vi "PH_ImageOperator.Best GAUSS Procedure.vi"(1 "Diameter":dbl, 2 "Data Trace":cluster{"Index":sgl[], "Trace":sgl[]}, 3 "calibrated?":bool, 4 "No Offset?":bool, 5 "error in (no error)":errorcluster) -> (16 "Best Fit Trace":cluster{"Index":sgl[], "Best Fit":dbl[]}, 17 "Best Fit Width Parameter":dbl, 18 "Best Fit Order":i32, 19 "error out":errorcluster)   [LabVIEW 2014, in "PH_ImageOperator.lvlib"]
doc: "Within this VI a GAUSS fit routine up to the 20th order is called and applied to the \"Data Trace\" (the Diameter\" is used within the fit routine as start value). The loop is stopped if the 10th order is reached or the mean square error increases. The error is caused by the fit routine only. If \"No Offset\" is true, within the fit function no offset is assumed."
uses:
  PH_ImageOperator.lvlib
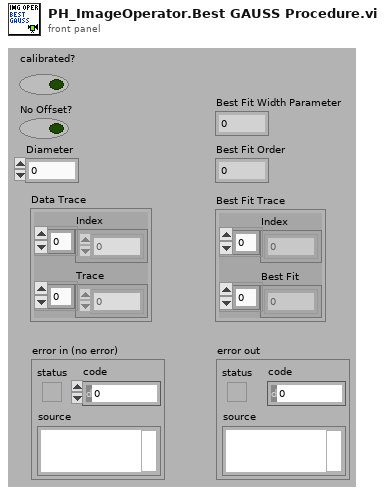
[diagram p1: front panel]
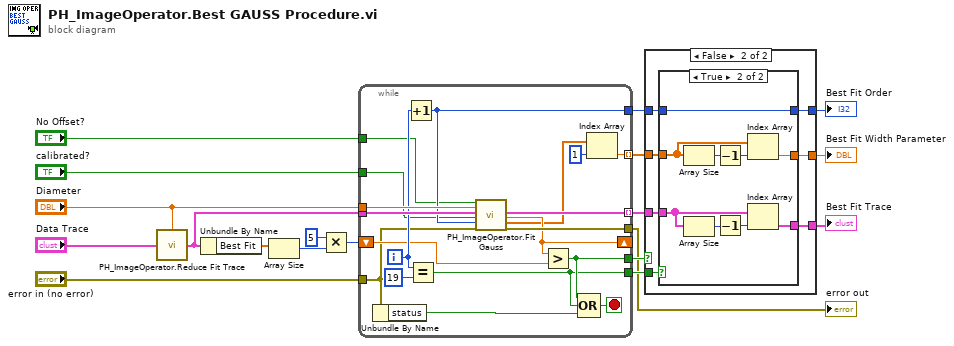
[diagram p0: block diagram]
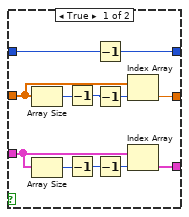
[diagram p2: hidden frame]
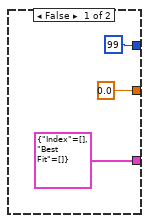
[diagram p3: hidden frame]
diagram:
  n1 = call "PH_ImageOperator.Reduce Fit Trace.vi"("Diameter"="Diameter", "Best Fit Trace"="Data Trace") -> ("Reduced Best Fit Trace"=w3:cluster{"Index":sgl[], "Best Fit":dbl[]})  [unwired: 13 in]
  n2 = Unbundle By Name(w3) -> ("Best Fit"=w9:dbl[])
  n3 = Array Size(array=w9) -> (size(s)=w6:i32)
  n4 = Multiply(x=5, y=w6) -> (x*y=w5:i32)
  n5 = while {
    tunnel: w3 -> [w38]
    tunnel: [w37] -> w17 mode=indexing
    tunnel: "Diameter" -> [w36]
    tunnel: "error in (no error)" -> [w24]
    tunnel: [w35] -> w11
    shift-right: [w34] -> _
    shift-left: w5 -> [w25]
    tunnel: [w30] -> w12
    tunnel: [w28] -> w13 mode=indexing
    tunnel: [w27] -> w16
    tunnel: [w26] -> w19
    tunnel: "calibrated?" -> [w22]
    tunnel: "No Offset?" -> [w20]
    i -> [w33]
    stop <- w31 stop-if-true
    n6 = Unbundle By Name(w24) -> ("status"=w23:bool)
    n7 = Increment(x=w33) -> (x+1=w30:i32)
    n8 = Equal?(x=w33, y=19) -> (x = y?=w26:bool)
    n9 = call "PH_ImageOperator.Fit Gauss.vi"("No Offset?"=w20, "Diam"=w36, "Trace"=w38, "calibrated?"=w22, "Order"=w30, "error in (no error)"=w24) -> ("Output"=w37:cluster{"Index":sgl[], "Best Fit":dbl[]}, "mse"=w34:dbl, "Best Fit Coefficients"=w21:dbl[], "error out"=w35:errorcluster)  [unwired: 10 in]
    n10 = Greater?(x=w34, y=w25) -> (0:w27:bool)
    n11 = Compound Arithmetic op=OR(w27, w26, w23) -> (w31:bool)
    n12 = Index Array(array=w21, index=1) -> (element=w28:dbl)
  }
  "error out" <- w11
  n13 = case shown="False" w16 {
    tunnel: w12 -> [w49 w51]
    tunnel: w13 -> [w47 w56]
    tunnel: [w50 w57] -> w14
    tunnel: [w48 w52] -> w15
    tunnel: w17 -> [w45 w55]
    tunnel: [w43 w54] -> w18
    tunnel: w19 -> [_ w53]
    frame True {
      n14 = Array Size(array=w47) -> (size(s)=w40:i32)
      n15 = Array Size(array=w45) -> (size(s)=w42:i32)
      n16 = Decrement(x=w40) -> (x-1=w39:i32)
      n17 = Decrement(x=w42) -> (x-1=w41:i32)
      n18 = Decrement(x=w49) -> (x-1=w48:i32)
      n19 = Decrement(x=w39) -> (x-1=w46:i32)
      n20 = Decrement(x=w41) -> (x-1=w44:i32)
      n21 = Index Array(array=w47, index=w46) -> (element=w50:dbl)
      n22 = Index Array(array=w45, index=w44) -> (element=w43:cluster{"Index":sgl[], "Best Fit":dbl[]})
    }
    frame False {
      n23 = case shown="True" w53 {
        tunnel: [0.0 ("Numeric") w69] -> w57
        tunnel: w56 -> [_ w68]
        tunnel: w55 -> [_ w64]
        tunnel: [cluster{"Index":sgl[], "Best Fit":dbl[]} {"Index"=[], "Best Fit"=[]} ("Output") w62] -> w54
        tunnel: [99 w61] -> w52
        tunnel: w51 -> [_ w61]
        frame False {
        }
        frame True {
          n24 = Array Size(array=w68) -> (size(s)=w67:i32)
          n25 = Array Size(array=w64) -> (size(s)=w65:i32)
          n26 = Decrement(x=w67) -> (x-1=w66:i32)
          n27 = Decrement(x=w65) -> (x-1=w63:i32)
          n28 = Index Array(array=w68, index=w66) -> (element=w69:dbl)
          n29 = Index Array(array=w64, index=w63) -> (element=w62:cluster{"Index":sgl[], "Best Fit":dbl[]})
        }
      }
    }
  }
  "Best Fit Trace" <- w18
  "Best Fit Order" <- w15
  "Best Fit Width Parameter" <- w14
